vi "Example.vi"(0 "GMap Options":cluster{"URL":T1, "Path":T2, "Marker":T3} {"URL"."Zoom" items=["World"=1, "Landmass/continent"=5, "City"=10, "Street"=15, "Building"=20]}, 5 "error in":errorcluster, 6 "Google Maps API Key":string, 12 "?":refnum<k7>(container)) -> (14 "Distance Matrix":cluster{"Duration":string, "Distance":string}, 15 "Geocode":cluster{"Latitude":string, "Longitude":string}, 16 "Elevation":cluster{"Elevation":string, "Resolution":string}, 17 "Time Zone":T4, 19 "error out":errorcluster)   [LabVIEW 2016]
doc: "GMaps API creates your map based on URL parameters sent through a standard HTTP request and returns the map as an image."
uses:
  Controls/URL.ctl
  Controls/Path.ctl
  Controls/Marker.ctl
  GMaps API.lvclass
panel:
  in  "stop":bool
  # "Instructions:\n1. To get a free Google Maps API Key go to https://console.developers.google.com.\n2. In URL define X and Y map parameters.\n3. Specify desired map parameters.\n4. Run the VI.\n5. Click Stop to stop the VI."
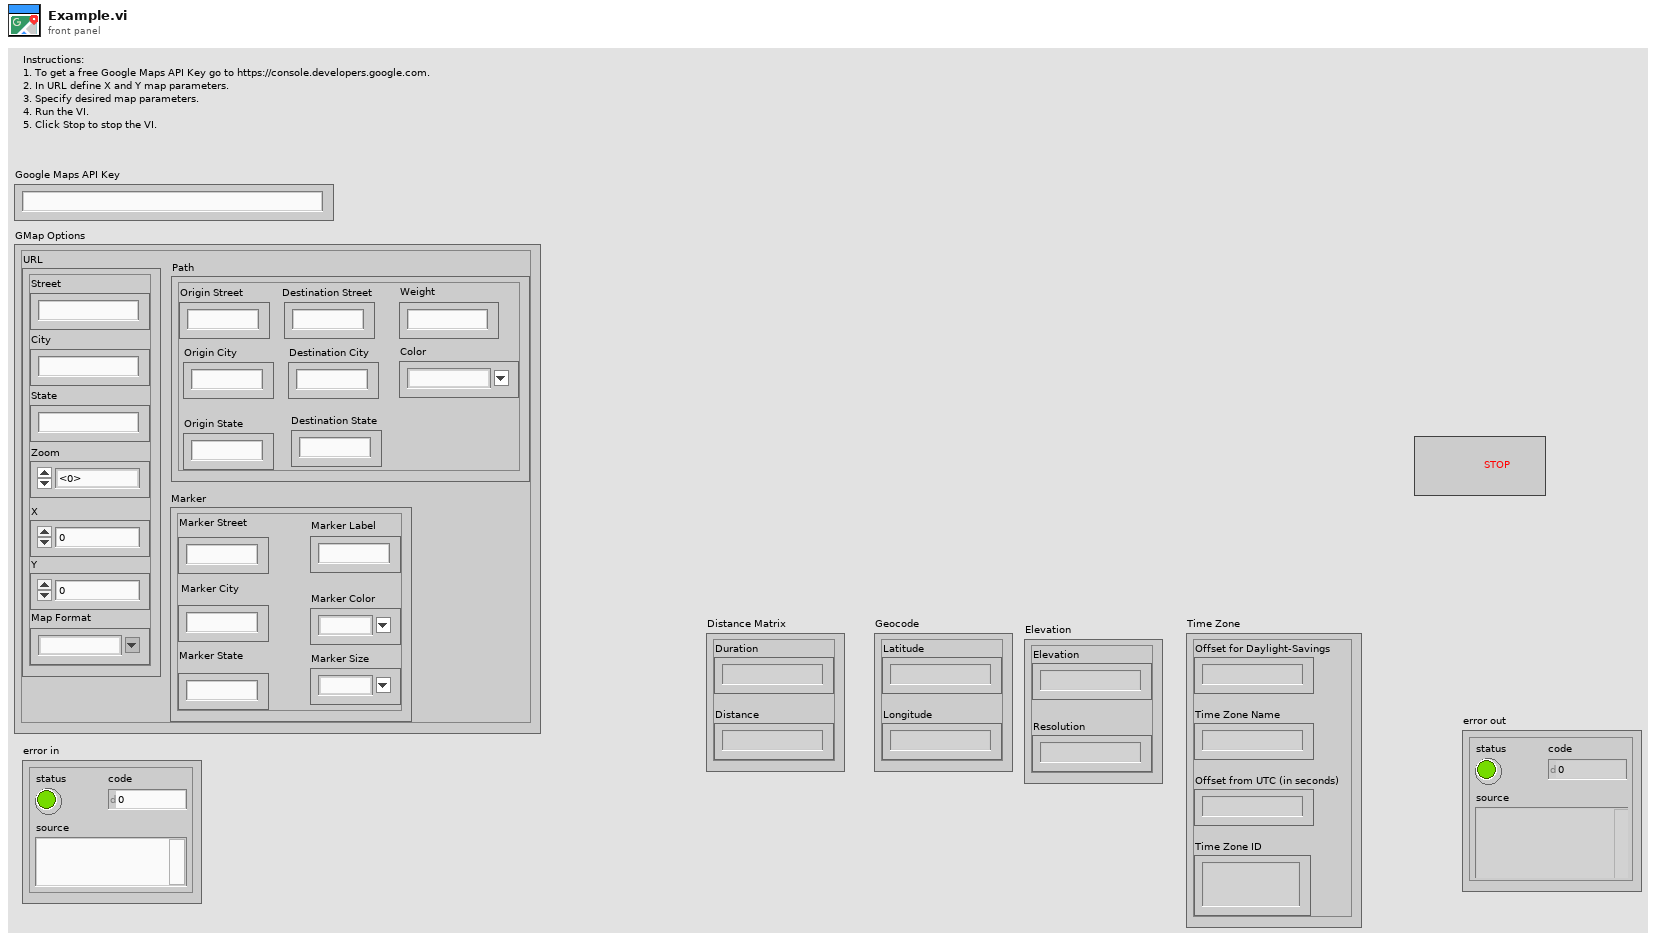
[diagram p1: front panel]
types:
  T1 = typedef "GMaps API.lvclass/URL.ctl" = cluster{"Street":string, "State":string, "City":string, "X":u32, "Y":u32, "Map Format":string, "Zoom":u64}
  T2 = typedef "GMaps API.lvclass/Path.ctl" = cluster{"Color":string, "Weight":string, "Destination State":string, "Destination City":string, "Destination Street":string, "Origin State":string, "Origin City":string, "Origin Street":string}
  T3 = typedef "GMaps API.lvclass/Marker.ctl" = cluster{"Marker Color":string, "Marker Size ":string, "Marker Label":string, "Marker State":string, "Marker City":string, "Marker Street":string}
  T4 = cluster{"Offset for Daylight-Savings":string, "Offset from UTC (in seconds)":string, "Time Zone Name":string, "Time Zone ID":string}
  T5 = cluster{"Distance Matrix":cluster{"Duration":string, "Distance":string}, "Time Zone":cluster{"Offset from UTC (in seconds)":string, "Offset for Daylight-Savings":string, "Time Zone Name":string, "Time Zone ID":string}, "Elevation":cluster{"Elevation":string, "Resolution":string}, "Geocode":cluster{"Latitude":string, "Longitude":string}}
  T6 = cluster{"Offset from UTC (in seconds)":string, "Offset for Daylight-Savings":string, "Time Zone Name":string, "Time Zone ID":string}
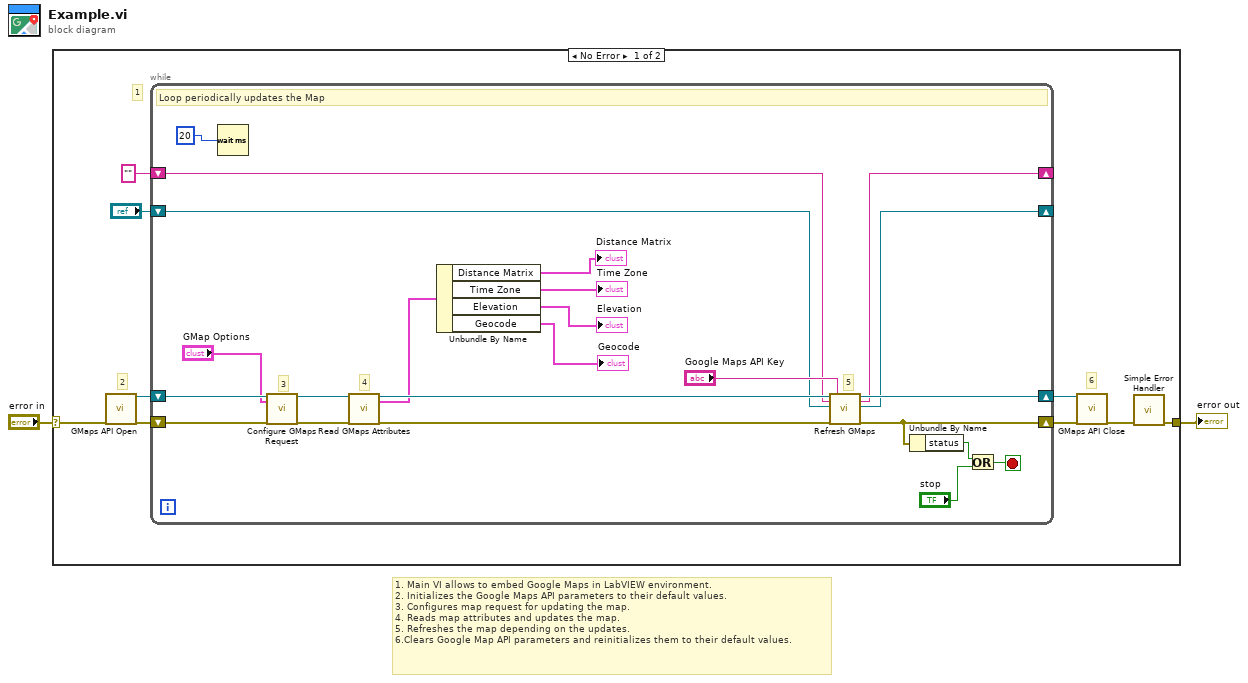
[diagram p0: block diagram]
diagram:
  # "1. Main VI allows to embed Google Maps in LabVIEW environment. \n2. Initializes the Google Maps API parameters to their default values.\n3. Configures map request for updating the map.\n4. Reads map attributes and updates the map.\n5. Refreshes the map depending on the updates.\n6.Clears Google Map API parameters and reinitializes them to their default values."
  n1 = case shown="No Error" "error in" {
    selector: "error in" -> [w4 w35]
    tunnel: [w3 w35] -> w1
    frame No Error {
      # "6"
      # "2"
      # "1"
      n2 = call "GMaps API Open.vi"("error in (no error)"=w4) -> ("GMaps API out"=w9:refnum<class "GMaps API.lvclass">, "error out"=w8:errorcluster)  [unwired: 17 in]
      n3 = while {
        shift-right: [w25] -> w7
        shift-left: w9 -> [w13]
        shift-right: [w23] -> w6
        shift-left: w8 -> [w14]
        shift-right: [w19] -> _
        shift-left: "?" -> [w18]
        shift-right: [w20] -> _
        shift-left: "" -> [w21]
        stop <- w31 stop-if-true
        # "5"
        # "4"
        # "3"
        # "Loop periodically updates the Map"
        n4 = Wait (ms)(milliseconds to wait=u32 20 ("millisecond multiple")) -> ()  [unwired: 1 out]
        n5 = call "Configure GMaps Request.vi"("GMaps API in"=w13, "GMap Options"="GMap Options", "error in (no error)"=w14) -> ("GMaps API out"=w16:refnum<class "GMaps API.lvclass">, "error out"=w15:errorcluster)  [unwired: 15 in]
        n6 = call "Read GMaps Attributes.vi"("GMaps API in"=w16, "error in (no error)"=w15) -> ("GMaps API out"=w26:refnum<class "GMaps API.lvclass">, "GMaps Attributes"=w17:T5, "error out"=w24:errorcluster)  [unwired: 15 in]
        n7 = Unbundle By Name(w17) -> ("Distance Matrix"=→"Distance Matrix":cluster{"Duration":string, "Distance":string}, "Time Zone"=→"Time Zone":T6, "Elevation"=→"Elevation":cluster{"Elevation":string, "Resolution":string}, "Geocode"=→"Geocode":cluster{"Latitude":string, "Longitude":string})
        n8 = call "Refresh GMaps.vi"("GMaps API in"=w26, "Updating String"=w21, "Automation Refnum in"=w18, "error in (no error)"=w24, "Google Maps API Key"="Google Maps API Key") -> ("GMaps API out"=w25:refnum<class "GMaps API.lvclass">, "Updated String"=w20:string, "Automation Refnum out"=w19:refnum<k7>, "error out"=w23:errorcluster)  [unwired: 11 in]
        n9 = Unbundle By Name(w23) -> ("status"=w33:bool)
        n10 = Or(x=w33, y="stop") -> (x .or. y?=w31:bool)
      }
      n11 = call "GMaps API Close.vi"("GMaps API in"=w7, "error in (no error)"=w6) -> ("error out"=w5:errorcluster)  [unwired: 16 in, 1 out]
      n12 = call <vilib>:"Simple Error Handler.vi"("error in (no error)"=w5) -> ("error out"=w3:errorcluster)  [unwired: 4 in, 4 out]
    }
    frame Error {
    }
  }
  "error out" <- w1
